vi "mmWave RX driver (FPGA).vi"() -> ()   [LabVIEW 2019]
uses:
  SubVIs/Sync/Sync Control.ctl
  SubVIs/Sync/Sync Measurements.ctl
  <instrlib>/_niInstr/DSP/v1/Shared/Public/IQ Impairments.ctl
  <instrlib>/_niInstr/DSP/v1/Shared/Public/Filter Coefficients.ctl
  Host/SubVIs/Low-level/TypeDefs/Gain Setting.ctl
  <instrlib>/niMmWave/ni3620/Config/v1/FPGA/Public/Typedefs/TX1 RX1 Port.ctl
  SubVIs/Utility/FPGA driver trigger source.ctl
  SubVIs/Utility/FPGA driver trigger destination.ctl
  <instrlib>/FlexRIO/DRAM FIFO/v2/FPGA/DRAM FIFO/DRAM FIFO Status.ctl
  <vilib>/Platform/TimedLoop/XDataNode/timing_clust.ctl
  <vilib>/Platform/TimedLoop/XDataNode/nitl_modes.ctl
  <vilib>/Platform/TimedLoop/XDataNode/wakeup.ctl
  <instrlib>/FlexRIO/DRAM FIFO/v2/FPGA/DRAM FIFO/FIFO Depth.ctl
  <instrlib>/FlexRIO/DRAM FIFO/v2/FPGA/DRAM FIFO/dynamic arbitration select.ctl
  <instrlib>/FlexRIO/DRAM FIFO/v2/FPGA/DRAM FIFO/Private/DRAM FIFO U512/Create 512x1 DRAM FIFO.vi
  <vilib>/rvi/Emulation/niFpgaSctlEmulationGetInTimedLoop.vi
  <vilib>/rvi/Emulation/niFpgaEmulationReportErrorSimple.vi
  <vilib>/rvi/Emulation/niFpgaGetClockAttributes.vi
  <vilib>/rvi/Emulation/niFpgaCriticalErrorInLSC.vi
  <vilib>/rvi/Emulation/niFpgaProcessEmulError.vi
  <vilib>/rvi/interface/RandomDataEmulation/nirviRandomDataMultiElementFPGAFIFO.vi
  <instcachedir>/0/nirviRandomDataMultiElementFPGAFIFO_1ED88BA00AC641F388A9B1FAA20E354D.lvgen/nirviRandomDataMultiElementFPGAFIFO_1ED88BA00AC641F388A9B1FAA20E354D_003.vi
  <vilib>/rvi/interface/RandomDataEmulation/niFpgaRandomDataHandleErrors.vi
  <vilib>/rvi/eio/common/nirviEmuTemplateMethod_errors.vi
  <instrlib>/_niInstr/Basic Elements/v1/FPGA/Private/Count Up U16.vi
  SubVIs/Misc/Globals.vi
  <instrlib>/_niInstr/Basic Elements/v1/FPGA/Private/Count Down U32.vi
  <instrlib>/FlexRIO/DRAM FIFO/v2/FPGA/DRAM FIFO/Pack Boolean Array.vi
  <instrlib>/_niInstr/Data Formatting/v1/FPGA/Private/Convert/FXP(+-,12,1) array to Boolean Array.vi
  <vilib>/rvi/DataTransferAndStorage/Container/Common/niFpgaContainerGetUniqueNameForEmu.vi
  <vilib>/rvi/DataTransferAndStorage/Container/Common/niFpgaContainerSetEmuInfo.vi
  <vilib>/rvi/eio/common/nirviEmuReportErrorAndStop.vi
  <vilib>/rvi/Emulation/niFpgaEmulationIsFPGAContextNoSignature.vi
  <vilib>/rvi/errors/niFpgaSetErrorForExecOnDevCompSimple.vi
  <vilib>/rvi/FIFO/Fifo_Resource/nirvififoEmulationSetSize.vi
  <vilib>/rvi/FIFO/Fifo_Resource/nirviFifoEmulationQueueMgr.vi
  <instcachedir>/0/nirviFifoEmulationQueueMgr_E5CAEC123FF24DC58D834DCA3CDAA9B5.lvgen/nirviFifoEmulationQueueMgr_E5CAEC123FF24DC58D834DCA3CDAA9B5_008.vi
  <vilib>/Utility/error.llb/Clear Errors.vi
  <vilib>/rvi/FIFO/Fifo_Resource/nirvififoEmulationCreateLock.vi
  <vilib>/rvi/FIFO/Fifo_Resource/nirvififoEmulationObtainLock.vi
  <vilib>/rvi/FIFO/Fifo_Resource/nirvififoEmulationReleaseLock.vi
  <vilib>/rvi/occurrence/nirviWaitOnOccurrenceBase.vi
  <vilib>/rvi/errors/nirviReportUnexpectedCaseInternalError.vi
  <vilib>/rvi/errors/nirviReportUnexpectedCaseInternalError (U32).vi
  <vilib>/rvi/FIFO/Fifo_Resource/nirvififoEmulationDetermineInputValidOut.vi
  <vilib>/Platform/TimedLoop/XDataNode/XDataNode.xnode
  <vilib>/rvi/DataTransferAndStorage/Container/XNode/niFpgaContainer.xnode
  <vilib>/rvi/interface/RandomDataEmulation/nirviRandomDataFpgaMultiElementTemplate.vi
  <vilib>/eio/EIONode/EIONode.xnode
  <vilib>/eio/EIOMethodNode/EIOMethodNode.xnode
  <vilib>/rvi/LocalResourceManager/LocalResourceManager.xnode
  <vilib>/rvi/FIFO/Fifo_Resource/nirvififoEmulationRead.vi
  <vilib>/rvi/FIFO/Fifo_Resource/nirvififoEmulationWrite.vi
  <vilib>/Platform/TimedLoop/XDataNode/XDNodeRunTimeDep.lvlib
  <instrlib>/_niInstr/Basic Elements/v1/FPGA/niInstr Basic Elements v1 FPGA.lvlib
  <instrlib>/niMmWave/ni3620/Config/v1/FPGA/niMmWave Config v1 FPGA.lvlib
  SubVIs/Utility/FPGA Utility.lvlib
  <instrlib>/FlexRIO/DRAM FIFO/v2/FPGA/DRAM FIFO/DRAM FIFO v2 FPGA.lvclass
  <instrlib>/_niInstr/Data Formatting/v1/FPGA/niInstr Data Formatting v1 FPGA.lvlib
  <instrlib>/FlexRIO/DRAM FIFO/v2/FPGA/DRAM FIFO/Private/DRAM FIFO U512/DRAM FIFO U512 v2 FPGA.lvclass
  <instrlib>/_niInstr/DSP/v1/Shared/niInstr DSP v1 Shared.lvlib
panel:
  out "dram.in fifo max":u32
  out "dram.highwater":u32
  out "dram.reset in progress?":bool
  in  "dram.reset":bool
  out "dram.status":T1
  out "dram.overflow":bool
  in  "dram.flush":bool
  out "acquisition active":bool
  out "aurora.data":u16
  out "aurora.trig count":u16
  out "pxi.trig count":u16
  out "aurora.tx val":u16
  in  "trig.pxi dst":i32
  in  "trig.export":T2
  in  "trig.export dur":u32
  in  "trig.source":T3
  out "debug.trig.count":u16
  in  "trig.delay":u16
  in  "trig.pxi src":i32
  in  "sync.master reset listen":bool
  in  "sync.counter reset enable":bool
  in  "20 kHz tclk parameters":T4
  out "tclk value":u16
  in  "gain ranging.enable port config":bool
  out "port 5.debug info":T5
  out "port 5.rx fifo overflow":bool
  in  "port 5.rx fifo overflow clear":bool
  in  "aurora.read port 5":bool
  out "port 4.rx fifo overflow":bool
  in  "port 4.rx fifo overflow clear":bool
  out "port 4.debug info":T5
  in  "aurora.read port 4":bool
  in  "gain ranging.enable coarse gain ranging":bool
  in  "gain ranging.enable fine gain ranging":bool
  in  "gain ranging.coarse gain values":fxp<+/-,16,12>[](array[numeric])=[0.0, 0.0, 0.0, 0.0]
  in  "table info":T6
  in  "gain ranging.manual setting":T9
  in  "gain ranging.setting list step":T10
  in  "gain ranging.enable":bool
  in  "gain ranging.dwell time (cycles)":u32=4800
  in  "rxjesd.control":T11
  out "rxjesd.status":T12
  in  "filter.enable":bool
  in  "filter.coefficients":T13
  in  "cal.correction":T15={"sample delay"={"I delay"=0.0, "Q delay"=0.0}, "fractional delay"={"enable"=FALSE, "coef write"=FALSE, "coef data"=0.0}, "impairments"={"inline gain I"=0.9999923706054688, "inline gain Q"=0.9999923706054688, "cross gain I"=0.0, "cross gain Q"=0.0, "pre-gain offset I"=0.0, "pre-gain offset Q"=0.0, "post-gain offset I"=0.0, "post-gain offset Q"=0.0}, "iq inversion"={"invert I"=FALSE, "invert Q"=FALSE}}
  out "sync.measurements":T16
  in  "sync.parameters":T18
  in  "acq.length":u32=1024
  out "aurora.fifo 1 overflow":bool
  in  "aurora.reset trigger":bool=TRUE
  out "aurora.fifo 0 overflow":bool
  in  "aurora.write":bool
  in  "aurora.fifo overflow clear":bool
  out "clocks valid":bool[](array[boolean])
  in  "cal.acquisition":T19={"acq length"=1024, "trigger type"=enum."software", "software trigger"=FALSE, "reset trigger detect"=FALSE}
  in  "sync.use synced trigger":bool
  in  "sync.trigger":bool
  # "DRAM and ACQUISITION"
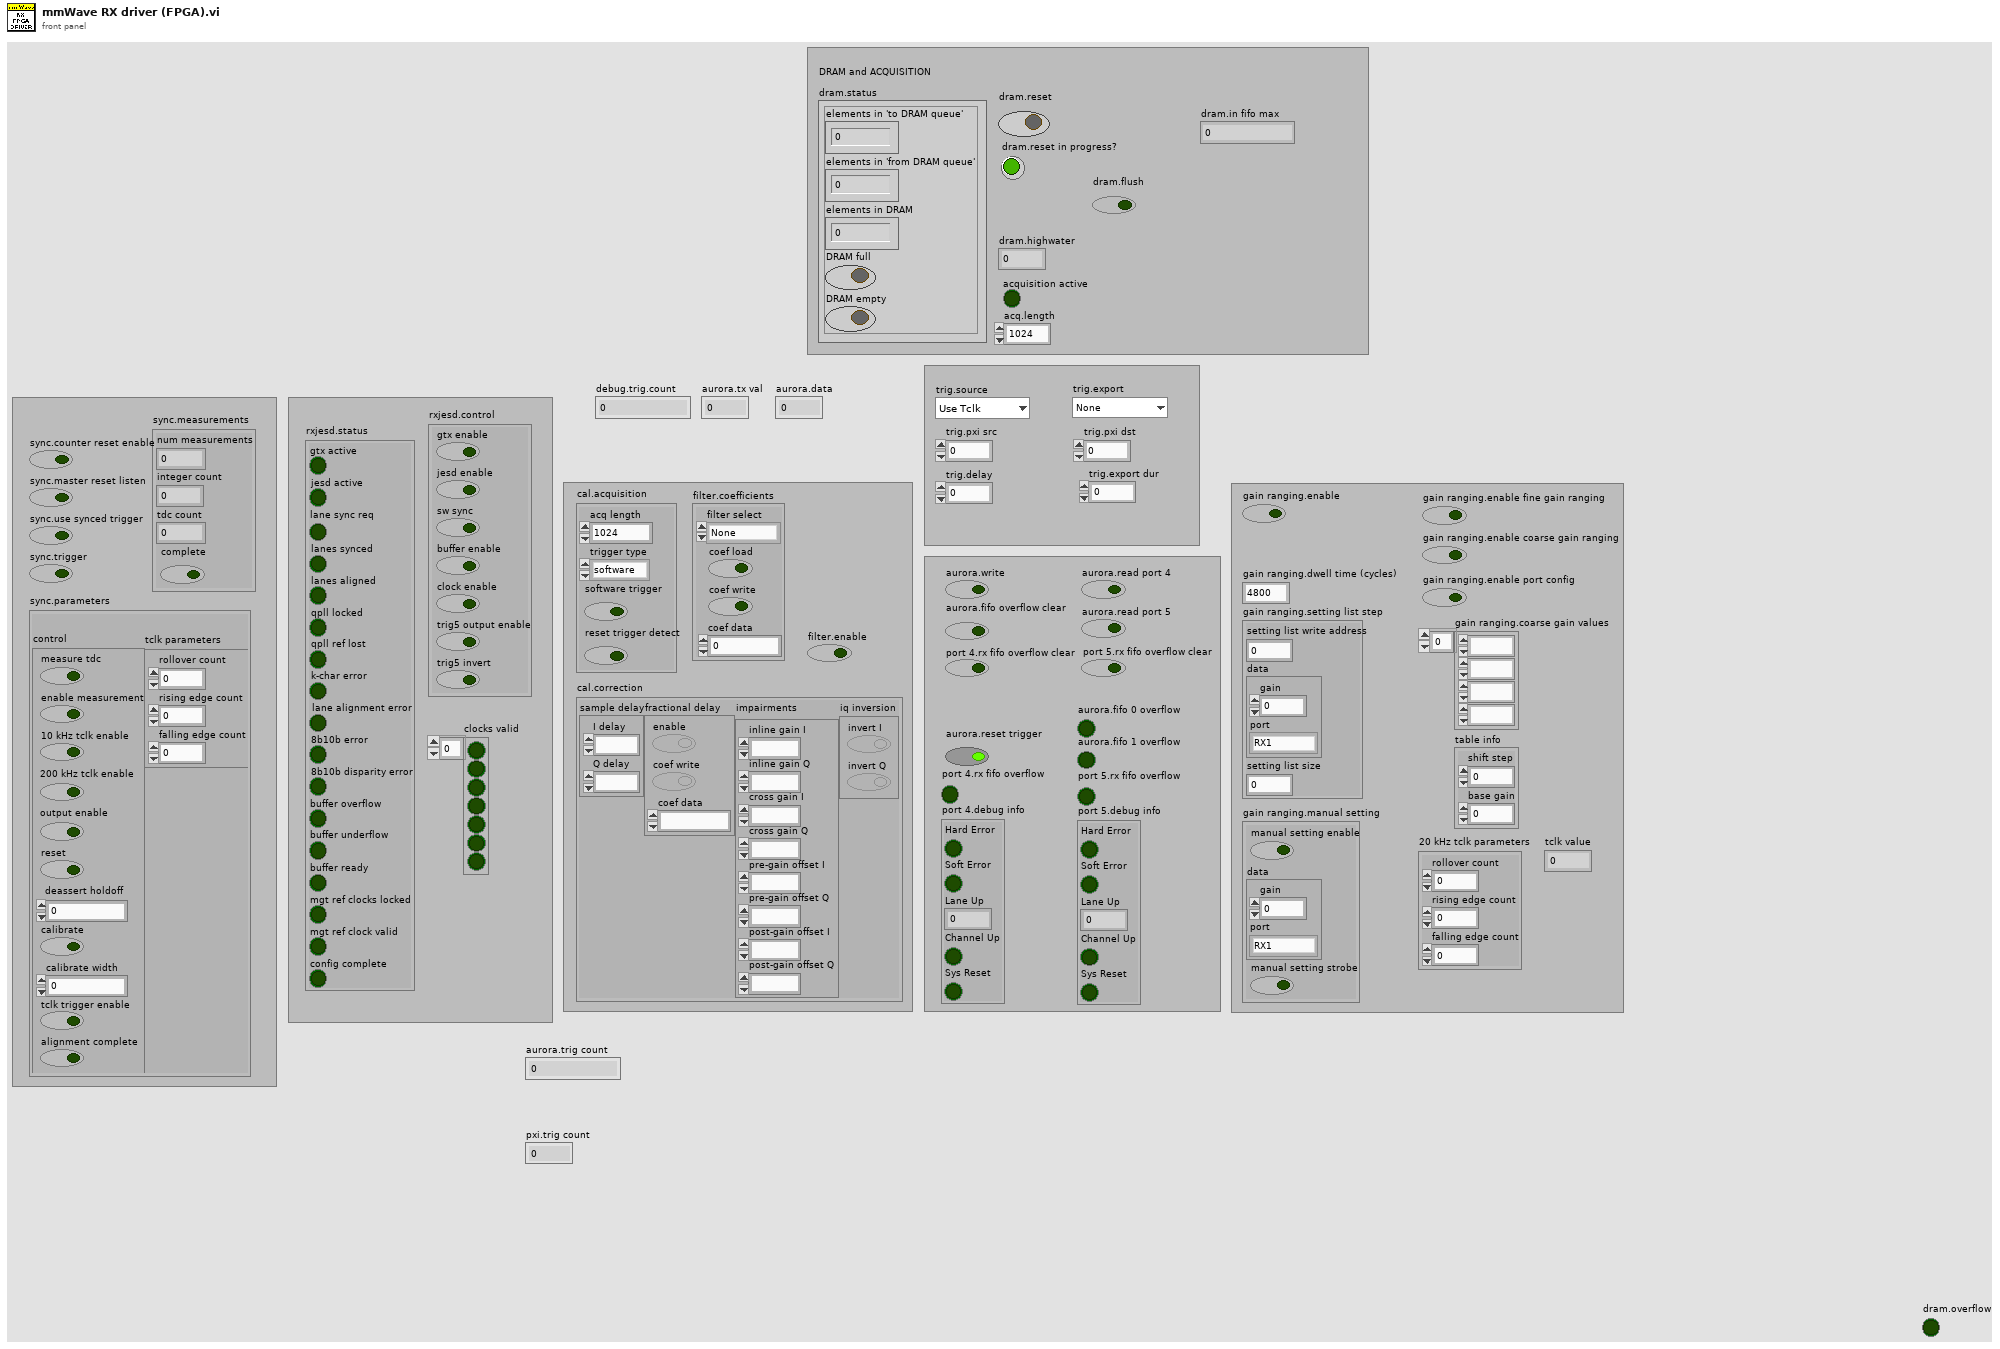
[diagram p1: front panel]
types:
  T1 = typedef "DRAM FIFO v2 FPGA.lvclass/DRAM FIFO Status.ctl" = cluster{"elements in 'to DRAM queue'":u32, "elements in 'from DRAM queue'":u32, "elements in DRAM":u32, "DRAM full":bool, "DRAM empty":bool}
  T2 = typedef "FPGA Utility.lvlib/FPGA driver trigger destination.ctl" = enum16{"None", "Source trig", "Synced trig", "Delayed sync"}
  T3 = typedef "FPGA Utility.lvlib/FPGA driver trigger source.ctl" = enum16{"Use Tclk", "PXI_Trig", "Aurora RX trig"}
  T4 = cluster{"rollover count":u16, "rising edge count":u16, "falling edge count":u16}
  T5 = cluster{"Hard Error":bool, "Soft Error":bool, "Lane Up":fxp<+,4,4>, "Channel Up":bool, "Sys Reset":bool}
  T6 = cluster{"shift step":i16, "base gain":fxp<+/-,16,12>}
  T7 = typedef "gain setting.ctl" = cluster{"gain":fxp<+/-,16,12>, "port":T8}
  T8 = typedef "TX1 RX1 Port.ctl" = enum8{"RX1", "TX1/RX2"}
  T9 = cluster{"manual setting enable":bool, "data":T7, "manual setting strobe":bool}
  T10 = cluster{"setting list write address":u32, "data":T7, "setting list size":u16}
  T11 = cluster{"gtx enable":bool, "jesd enable":bool, "sw sync":bool, "buffer enable":bool, "clock enable":bool, "trig5 output enable":bool, "trig5 invert":bool}
  T12 = cluster{"gtx active":bool, "jesd active":bool, "lane sync req":bool, "lanes synced":bool, "lanes aligned":bool, "qpll locked":bool, "qpll ref lost":bool, "k-char error":bool, "lane alignment error":bool, "8b10b error":bool, "8b10b disparity error":bool, "buffer overflow":bool, "buffer underflow":bool, "buffer ready":bool, "mgt ref clocks locked":bool, "mgt ref clock valid":bool, "config complete":bool}
  T13 = typedef "niInstr DSP v1 Shared.lvlib/Filter Coefficients.ctl" = cluster{"filter select":enum8{"None", "I Inline", "I Cross", "Q Cross", "Q Inline"}, "coef load":bool, "coef write":bool, "coef data":fxp<+/-,18,1>}
  T14 = typedef "niInstr DSP v1 Shared.lvlib/IQ Impairments.ctl" = cluster{"inline gain I":fxp<+/-,18,1>, "inline gain Q":fxp<+/-,18,1>, "cross gain I":fxp<+/-,18,1>, "cross gain Q":fxp<+/-,18,1>, "pre-gain offset I":fxp<+/-,18,1>, "pre-gain offset Q":fxp<+/-,18,1>, "post-gain offset I":fxp<+/-,18,1>, "post-gain offset Q":fxp<+/-,18,1>}
  T15 = cluster{"sample delay":cluster{"I delay":fxp<+,13,13>, "Q delay":fxp<+,13,13>}, "fractional delay":cluster{"enable":bool, "coef write":bool, "coef data":fxp<+/-,18,1>}, "impairments":T14, "iq inversion":cluster{"invert I":bool, "invert Q":bool}}
  T16 = typedef "Sync Measurements.ctl" = cluster{"num measurements":u16, "integer count":u16, "tdc count":u16, "complete":bool}
  T17 = typedef "Sync Control.ctl" = cluster{"measure tdc":bool, "enable measurement":bool, "10 kHz tclk enable":bool, "200 kHz tclk enable":bool, "output enable":bool, "reset":bool, "deassert holdoff":u8, "calibrate":bool, "calibrate width":u8, "tclk trigger enable":bool, "alignment complete":bool}
  T18 = cluster{"control":T17, "tclk parameters":cluster{"rollover count":u16, "rising edge count":u16, "falling edge count":u16}}
  T19 = cluster{"acq length":u16, "trigger type":enum16{"software", "external", "rising zero", "falling zero"}, "software trigger":bool, "reset trigger detect":bool}
  T20 = typedef "DRAM FIFO v2 FPGA.lvclass/FIFO Depth.ctl" = u8
  T21 = cluster{"m_axis_tvalid":refnum<k21>, "m_axis_tdata_0":refnum<k21>, "m_axis_tdata_1":refnum<k21>, "m_axis_tdata_2":refnum<k21>, "m_axis_tdata_3":refnum<k21>}
  T22 = cluster{"s_axis_tvalid":refnum<k21>, "s_axis_tdata_0":refnum<k21>, "s_axis_tdata_1":refnum<k21>, "s_axis_tdata_2":refnum<k21>, "s_axis_tdata_3":refnum<k21>, "s_axis_tready":refnum<k21>}
  T23 = typedef "XDNodeRunTimeDep.lvlib/timing_clust.ctl" = cluster{"Expected End [f-1]":u64, "Actual End [f-1]":u64, "Finished Late? [f-1]":bool, "Expected End [i-1]":u64, "Actual End [i-1]":u64, "Finished Late? [i-1]":bool, "Expected Start [i]":u64, "Actual Start [i]":u64, "Expected Start [f]":u64, "Actual Start [f]":u64, "Source Name":string, "Structure Name":string, "Period":i64, "Deadline":i64, "Offset":i64, "Start":i64, "Priority":i32, "Timeout":i32, "Mode":T24, "Wakeup Reason":T25, "Error":errorcluster, "Source Type":string, "Secondary Source Type":string, "Global End Time":u64, "Global Start Time":u64, "Frame Duration":u64, "Iteration Duration":u64, "Assigned CPU":i32, "I/O Scan Engine Mode":u32}
  T24 = typedef "XDNodeRunTimeDep.lvlib/nitl_modes.ctl" = enum32{"No Change", "Process missed periods, maintain original phase", "Discard missed periods, maintain original phase", "Process missed periods, ignore original phase", "Discard missed periods, ignore original phase"}
  T25 = typedef "XDNodeRunTimeDep.lvlib/wakeup.ctl" = enum32{"Normal", "Aborted", "Asynchronous wakeup", "Timing source error", "Timed loop error", "Timeout"}
  T26 = typedef "Sync Resources.ctl" = cluster{"tdc assert":refnum<k21>, "tdc deassert":refnum<k21>, "tdc count":refnum<k21>, "control":refnum<k21>, "integer count":refnum<k21>}
  T27 = typedef "DRAM FIFO v2 FPGA.lvclass/dynamic arbitration select.ctl" = enum16{"none", "dynamic (priority writes)", "dynamic (priority reads)"}
  T28 = cluster{"disable TClk measure":bool, "output enable":bool, "output value":bool}
  T29 = typedef "niInstr DSP v1 Shared.lvlib/IQ Data.ctl" = cluster{"I":fxp<+/-,18,1>, "Q":fxp<+/-,18,1>, "overflow":bool}
  T30 = typedef "AXI4-Stream Reader FXP64x4 Resources.ctl" = cluster{"AXI4-Stream Reader Resources":cluster{"Use TREADY":bool, "Use TLAST":bool, "TLAST":refnum<k21>, "TREADY":refnum<k21>, "TVALID":refnum<k21>, "Use TKEEP":bool, "Use TSTRB":bool, "Use TUSER":bool}, "TDATA Resources":cluster{"TDATA_0":refnum<k21>, "TDATA_1":refnum<k21>, "TDATA_2":refnum<k21>, "TDATA_3":refnum<k21>}, "TKEEP":refnum<k21>, "TSTRB":refnum<k21>}
  T31 = typedef "AXI4-Stream Writer FXP64x4 Resources.ctl" = cluster{"Writer Resources":cluster{"Use TREADY":bool, "Use TLAST":bool, "TLAST":refnum<k21>, "TREADY":refnum<k21>, "TVALID":refnum<k21>, "Use TSTRB":bool, "Use TKEEP":bool, "Use TUSER":bool}, "TDATA Resources":cluster{"TDATA_0":refnum<k21>, "TDATA_1":refnum<k21>, "TDATA_2":refnum<k21>, "TDATA_3":refnum<k21>}, "TKEEP":refnum<k21>, "TSTRB":refnum<k21>}
  T32 = cluster{"Hard Error":refnum<k21>, "Soft Error":refnum<k21>, "Lane Up":refnum<k21>, "Channel Up":refnum<k21>, "Sys Reset":refnum<k21>}
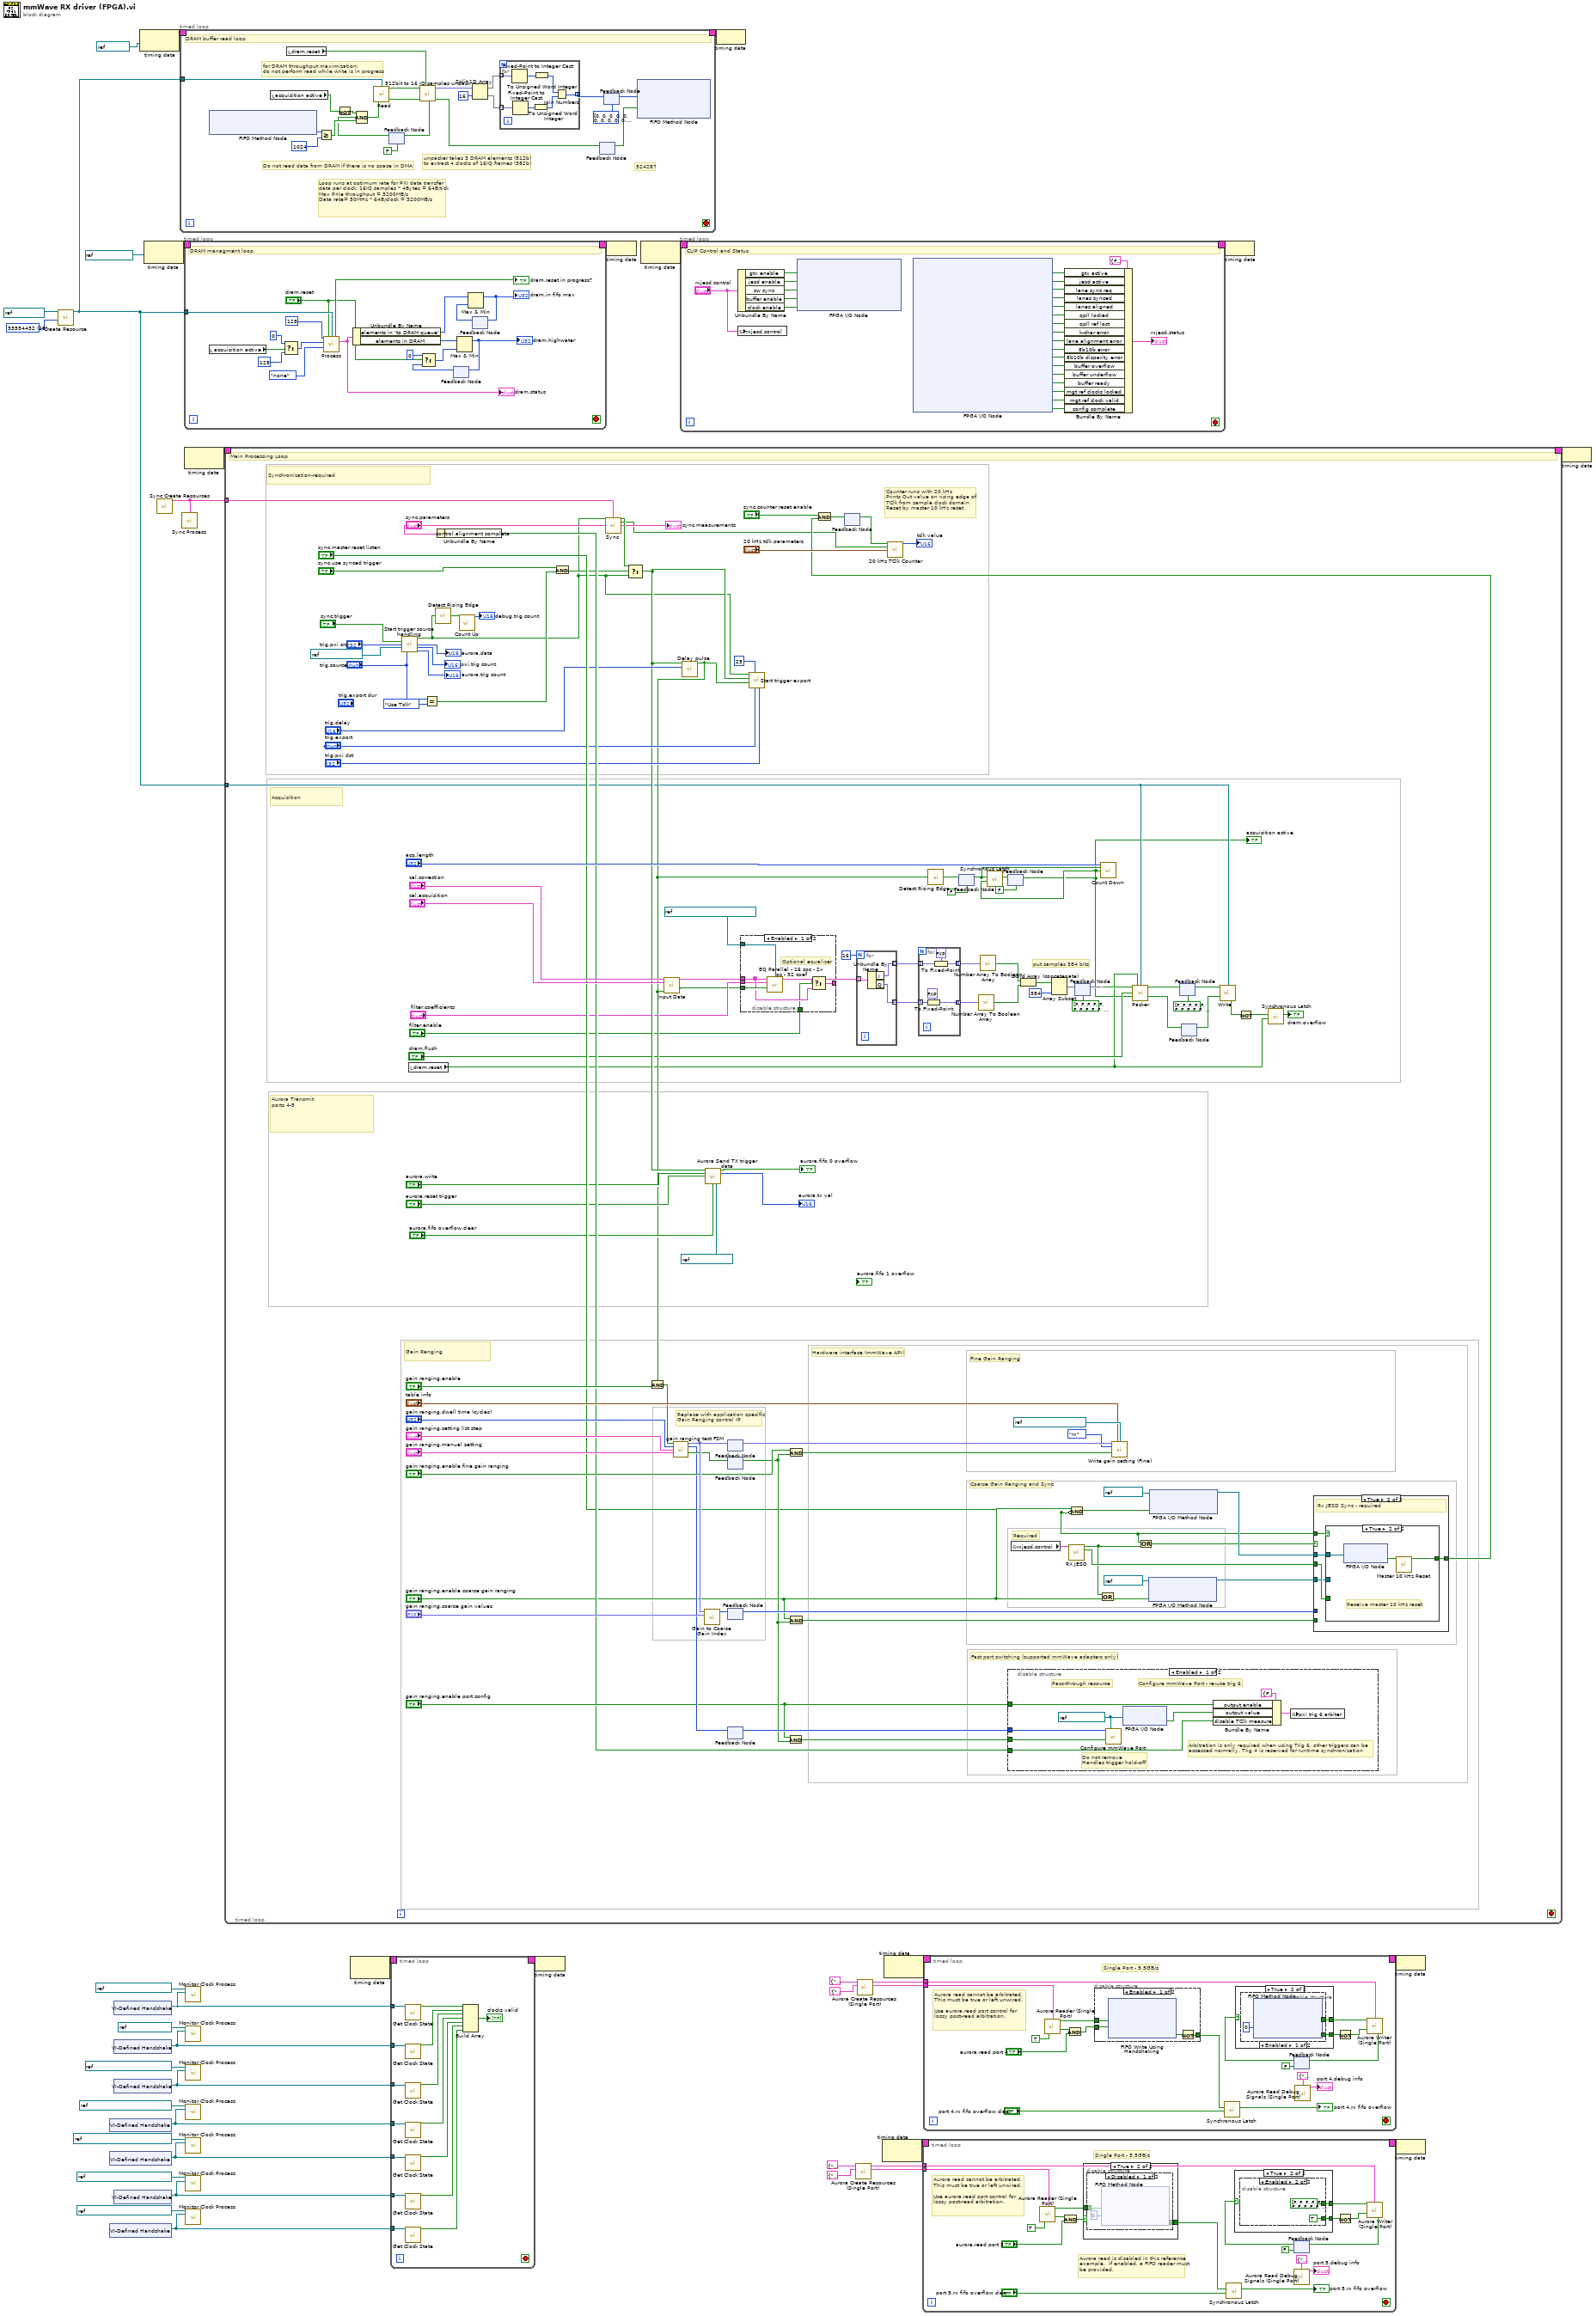
[diagram p0: block diagram]
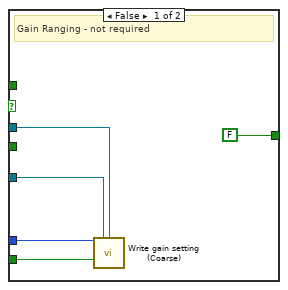
[diagram p3: hidden frame]
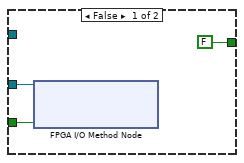
[diagram p4: hidden frame]
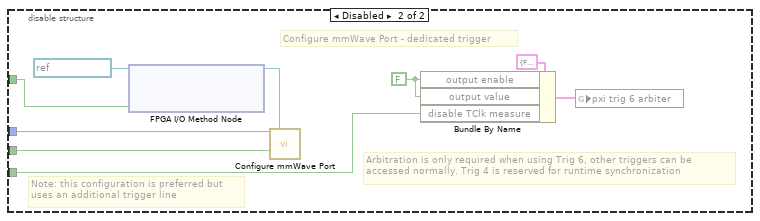
[diagram p5: hidden frame]
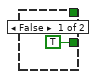
[diagram p6: hidden frame]
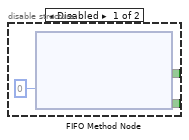
[diagram p7: hidden frame]
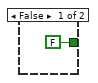
[diagram p8: hidden frame]
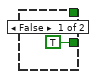
[diagram p11: hidden frame]
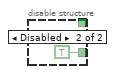
[diagram p12: hidden frame]
diagram:
  w1 = T20 25 items=["4"=2, "8"=3, "16"=4, "32"=5, "64"=6, "128"=7, "256"=8, "512"=9, "1024"=10, "2048"=11, "4096"=12, "8192"=13, "16384"=14, "32768"=15, "65536"=16, "131072"=17, "262144"=18, "524288"=19, "1048576"=20, "2097152"=21, "4194304"=22, "8388608"=23, "16777216"=24, "33554432"=25, "67108864"=26, "134217728"=27, "268435456"=28, "536870912"=29, "1073741824"=30, "2147483648"=31, "4294967296"=32] ("actual # of DRAM elements")
  n1 = call-poly <instrlib>:"Create Resource.vi"("actual # of DRAM elements"=w1, "memory refnum"=refnum<k21> "RX memo") -> ("DRAM FIFO ref out"=w2:refnum<class "DRAM FIFO v2 FPGA.lvclass">)  [unwired: 9 in]
  n2 = xnode "VI-Defined Handshake"() -> ("Handshake Out"=w19:refnum<k21>)
  n3 = xnode "VI-Defined Handshake"() -> ("Handshake Out"=w20:refnum<k21>)
  n4 = xnode "VI-Defined Handshake"() -> ("Handshake Out"=w27:refnum<k21>)
  n5 = xnode "VI-Defined Handshake"() -> ("Handshake Out"=w34:refnum<k21>)
  n6 = xnode "VI-Defined Handshake"() -> ("Handshake Out"=w33:refnum<k21>)
  n7 = xnode "VI-Defined Handshake"() -> ("Handshake Out"=w29:refnum<k21>)
  n8 = xnode "VI-Defined Handshake"() -> ("Handshake Out"=w30:refnum<k21>)
  n9 = node-c288(refnum<k21> "50MHz" ("Source Name")) -> (w5:T23)
  n10 = node-c288(refnum<k21> "DRAM Clock" ("Source Name")) -> (w8:T23)
  n11 = call "Sync Create Resources.vi"() -> ("sync.resources"=w38:T26)  [unwired: 15 in]
  n12 = timed-loop {
    timing: w5 -> [_]
    timing-out: [_] -> w4
    tunnel: w2 -> [w46]
    stop <- _ stop-if-true
    # "524287"
    # "unpacker takes 3 DRAM elements (512b)\nto extract 4 clocks of 16IQ frames (382b)"
    # "Do not read data from DRAM if there is no space in DMA"
    # "for DRAM throughput maximization:\ndo not perform read while write is in progress"
    # "Loop runs at optimum rate for PXI data transfer\ndata per clock: 16IQ samples * 4Bytes = 64B/tick\nMax PXIe throughput = 3200MB/s\nData rate= 50MHz * 64B/clock = 3200MB/s"
    # "DRAM buffer read loop"
    n13 = xnode ("FIFO Method Node")() -> ("Number of Elements to Write"=w57:u32)  [unwired: 1 in, 1 out]
    n14 = local read "acquisition active"() -> (w45:bool)
    n15 = local read "dram.reset"() -> (w43:bool)
    n16 = Greater Or Equal?(x=w57, y=u32 1024) -> (x >= y?=w59:bool)
    n17 = Not(x=w45) -> (.not. x?=w48:bool)
    n18 = feedback #1(FALSE ("ready for input")) -> (w49:bool)
    n19 = Compound Arithmetic op=AND(w48, w49, w59) -> (w50:bool)
    n20 = call <instrlib>:"Read.vi"("DRAM FIFO ref in"=w46, "ready for output"=w50) -> ("element"=w51:bool[], "output valid"=w52:bool)  [unwired: 12 in]
    n21 = call "512bit to 16 IQ samples unpack.vi"("reset"=w43, "input valid"=w52, "data in"=w51) -> ("output valid"=w63:bool, "data out"=w54:fxp<+/-,12,1>[], "ready for input"=w53:bool)  [unwired: 6 in]
    n22 = feedback-in #1(w53) -> ()
    n23 = Split 1D Array(array=w54, index=16) -> (first subarray=w55:fxp<+/-,12,1>[], second subarray=w56:fxp<+/-,12,1>[])
    n24 = for {
      tunnel: w55 -> [w71] mode=indexing
      tunnel: w56 -> [w70] mode=indexing
      tunnel: [w67] -> w60 mode=indexing
      n25 = Fixed-Point to Integer Cast(1:w71) -> (0:w66:i16)
      n26 = Fixed-Point to Integer Cast(1:w70) -> (0:w65:i16)
      n27 = To Unsigned Word Integer(number=w65) -> (unsigned 16bit integer=w68:u16)
      n28 = To Unsigned Word Integer(number=w66) -> (unsigned 16bit integer=w69:u16)
      n29 = Join Numbers(hi=w69, lo=w68) -> ((hi.lo)=w67:u32)
    }
    n30 = feedback #2() -> (w64:bool)  [unwired: 1 in]
    n31 = feedback-in #2(w63) -> ()
    n32 = feedback #3(u32[] [0, 0, 0, 0, 0, 0, 0, 0, 0, 0, 0, 0, 0, 0, 0, 0]) -> (w61:u32[])
    n33 = feedback-in #3(w60) -> ()
    n34 = xnode ("FIFO Method Node")("Element"=w61, "Input Valid"=w64) -> ()  [unwired: 1 in, 2 out]
  }
  n35 = call "Sync Process.vi"("sync.resources"=w38) -> ()  [unwired: 15 in]
  n36 = timed-loop {
    timing: w8 -> [_]
    timing-out: [_] -> w7
    tunnel: w2 -> [w85]
    stop <- _ stop-if-true
    # "DRAM managment loop"
    n37 = local read "acquisition active"() -> (w78:bool)
    n38 = Select(t=u16 0, s=w78, f=u16 128 ("read grant time (clock ticks)")) -> (s? t:f=w76:u16)
    n39 = call <instrlib>:"Process.vi"("write grant time (clock ticks)"=u16 128, "reset DRAM"="dram.reset", "DRAM FIFO ref in"=w85, "read grant time (clock ticks)"=w76, "dynamic arbitration"=dynamic_arbitration_select."none") -> ("reset in progress?"=→"dram.reset in progress?":bool, "status"=w88:T1)  [unwired: 9 in]
    "dram.status" <- w88
    n40 = Unbundle By Name(w88) -> ("elements in 'to DRAM queue'"=w80:u32, "elements in DRAM"=w87:u32)
    n41 = feedback #4() -> (w83:u32)  [unwired: 1 in]
    n42 = Select(t=u32 0, s="dram.reset", f=w83) -> (s? t:f=w81:u32)
    n43 = Max & Min(x=w87, y=w81) -> (max(x,y)=w86:u32)  [unwired: 1 out]
    "dram.highwater" <- w86
    n44 = feedback-in #4(w86) -> ()
    n45 = feedback #5() -> (w79:u32)  [unwired: 1 in]
    n46 = Max & Min(x=w80, y=w79) -> (max(x,y)=w74:u32)  [unwired: 1 out]
    "dram.in fifo max" <- w74
    n47 = feedback-in #5(w74) -> ()
  }
  n48 = node-c288() -> (w40:T23)  [unwired: 1 in]
  n49 = call "Monitor Clock Process.vi"("clock name"=refnum<k21> "40 MHz Onboard Clock", "handshake"=w34) -> ()  [unwired: 14 in]
  n50 = call "Monitor Clock Process.vi"("clock name"=refnum<k21> "100 MHz Clock", "handshake"=w33) -> ()  [unwired: 14 in]
  n51 = call "Monitor Clock Process.vi"("clock name"=refnum<k21> "7902R IO Socket\\SampleClk", "handshake"=w29) -> ()  [unwired: 14 in]
  n52 = call "Monitor Clock Process.vi"("clock name"=refnum<k21> "7902R IO Socket\\SampleClkx2", "handshake"=w19) -> ()  [unwired: 14 in]
  n53 = call "Monitor Clock Process.vi"("clock name"=refnum<k21> "7902R IO Socket\\SampleClkDiv2", "handshake"=w20) -> ()  [unwired: 14 in]
  n54 = call "Monitor Clock Process.vi"("clock name"=refnum<k21> "7902R IO Socket\\Port4_UserClk", "handshake"=w30) -> ()  [unwired: 14 in]
  n55 = call "Monitor Clock Process.vi"("clock name"=refnum<k21> "7902R IO Socket\\Port5_UserClk", "handshake"=w27) -> ()  [unwired: 14 in]
  n56 = timed-loop {
    timing: w40 -> [_]
    timing-out: [_] -> w39
    tunnel: w38 -> [w196]
    tunnel: w2 -> [w110]
    stop <- _ stop-if-true
    # "put samples 384 bits"
    # "Counter runs with 20 kHz\nPrints Out value on rising edge of \nTClk from sample clock domain\nReset by master 10 kHz reset"
    # "Replace with application specific Gain Ranging control IP"
    # "Fast port switching (supported mmWave adapters only)"
    # "Coarse Gain Ranging and Sync"
    # "Fine Gain Ranging"
    # "Hardware interface (mmWave API)"
    # "Gain Ranging"
    # "Aurora Transmit\nports 4-5"
    # "Acquisition"
    # "Synchronization-required"
    # "Required"
    # "Main Processing Loop"
    n57 = call "Start trigger source handling.vi"("sync.trigger"="sync.trigger", "trig.pxi trig src"="trig.pxi src", "Refnum in"=refnum<k21> "aurora rx fifo 0" ("FIFO In"), "trig.source"="trig.source") -> ("trigger"=w126:bool, "aurora.data"=→"aurora.data":u16, "pxi.trig count"=→"pxi.trig count":u16, "aurora.trig count"=→"aurora.trig count":u16)  [unwired: 8 in]
    n58 = local read "dram.reset"() -> (w100:bool)
    n59 = Equal?(x="trig.source", y=FPGA_driver_trigger_source."Use Tclk") -> (x = y?=w128:bool)
    n60 = call <instrlib>:"Detect Rising Edge.vi"("signal"=w126) -> ("edge detected"=w148:bool)  [unwired: 14 in]
    n61 = Unbundle By Name("sync.parameters") -> ("control.alignment complete"=w162:bool)
    n62 = call-poly <instrlib>:"Count Up.vi"("increment"=w148) -> ("count out"=→"debug.trig.count":u16)  [unwired: 14 in]
    n63 = And(x="sync.use synced trigger", y=w128) -> (x .and. y?=w129:bool)
    n64 = call "Sync.vi"("trigger"=w126, "sync.resources"=w196, "sync.parameters"="sync.parameters") -> ("synced trigger"=w197:bool, "tclk"=w153:bool, "sync measurements"=→"sync.measurements":T16)  [unwired: 10 in]
    n65 = Select(t=w197, s=w129, f=w126) -> (s? t:f=w140:bool)
    n66 = call "Delay pulse.vi"("delay"="trig.delay", "signal in"=w140) -> ("delayed rising edge"=w125:bool)  [unwired: 9 in]
    n67 = And(x=w125, y="gain ranging.enable") -> (x .and. y?=w177:bool)
    n68 = call "Input Data.vi"("cal parameters"="cal.correction", "acq parameters"="cal.acquisition", "external trigger"=w125) -> ("adc data"=w98:T29[], "output valid"=w94:bool)  [unwired: 11 in]
    n69 = call "gain ranging test FSM.vi"("gain ranging.start sequence"=w177, "gain ranging.dwell time (cycles)"="gain ranging.dwell time (cycles)", "gain ranging.gain setting list"="gain ranging.setting list step", "gain ranging.manual request"="gain ranging.manual setting") -> ("gain ranging.gain setting"=w186:fxp<+/-,16,12>, "gain ranging.TX1/RX1 Port Value"=w179:T8, "gain ranging.gain setting valid"=w181:bool)  [unwired: 8 in, 1 out]
    n70 = call "Gain to Coarse Gain Index.vi"("gain setting"=w186, "coarse gain values"="gain ranging.coarse gain values") -> ("coarse gain index"=w184:u32)  [unwired: 13 in]
    n71 = call "Aurora Send TX trigger data.vi"("start trigger"=w140, "aurora.write"="aurora.write", "aurora.reset trigger"="aurora.reset trigger", "clear overflow"="aurora.fifo overflow clear", "aurora tx fifo"=refnum<k21> "aurora tx fifo 0" ("FIFO In")) -> ("tx overflow latch"=→"aurora.fifo 0 overflow":bool, "trig count"=→"aurora.tx val":u16)  [unwired: 9 in]
    n72 = feedback #6() -> (w185:fxp<+/-,16,12>)  [unwired: 1 in]
    n73 = feedback-in #6(w186) -> ()
    n74 = feedback #7() -> (w167:bool)  [unwired: 1 in]
    n75 = feedback-in #7(w181) -> ()
    n76 = feedback #8() -> (w170:u32)  [unwired: 1 in]
    n77 = feedback-in #8(w184) -> ()
    n78 = feedback #9() -> (w175:T8)  [unwired: 1 in]
    n79 = feedback-in #9(w179) -> ()
    n80 = disable-structure shown="Enabled" {
      disable-tunnel: w94 -> [w211 _]
      disable-tunnel: [w209 w212] -> w97
      disable-tunnel: w98 -> [w208 w212]
      disable-tunnel: "filter.coefficients" -> [w207 _]
      disable-tunnel: "filter.enable" -> [w206 _]
      disable-tunnel: refnum<k21> "7902R IO Socket\\SampleClkx2" ("clock x2") -> [w205 _]
      frame Enabled {
        # "Optional equalizer"
        n81 = call "EQ Parallel - 16 spc - 2x oc - 32 coef.vi"("data in"=w208, "clock x2"=w205, "filter coefficients"=w207, "input valid"=w211) -> ("data out"=w210:T29[])  [unwired: 9 in, 2 out]
        n82 = Select(t=w210, s=w206, f=w208) -> (s? t:f=w209:T29[])
      }
      frame Disabled {
      }
    }
    n83 = call "Start trigger export.vi"("trig.pxi trig dst"="trig.pxi dst", "trig.export"="trig.export", "trig.dur"=u32 25, "delayed trigger"=w125, "synced trigger"=w140, "source trigger"=w126) -> ()  [unwired: 2 in, 4 out]
    n84 = And(x="gain ranging.enable port config", y=w167) -> (x .and. y?=w166:bool)
    n85 = And(x="gain ranging.enable fine gain ranging", y=w167) -> (x .and. y?=w180:bool)
    n86 = And(x="gain ranging.enable coarse gain ranging", y=w167) -> (x .and. y?=w169:bool)
    n87 = feedback #10() -> (w154:bool)  [unwired: 1 in]
    n88 = for {
      N: 16 -> [_]
      tunnel: w97 -> [w221] mode=indexing
      tunnel: [w220] -> w103 mode=indexing
      tunnel: [w219] -> w106 mode=indexing
      n89 = Unbundle By Name(w221) -> ("I"=w220:fxp<+/-,18,1>, "Q"=w219:fxp<+/-,18,1>)
    }
    n90 = call "20 kHz TClk Counter.vi"("master 10 kHz reset"=w154, "tclk"=w153, "20 kHz tclk parameters"="20 kHz tclk parameters") -> ("tclk offset value"=→"tclk value":u16)  [unwired: 12 in]
    n91 = for {
      tunnel: w103 -> [w215] mode=indexing
      tunnel: w106 -> [w217] mode=indexing
      tunnel: [w214] -> w105 mode=indexing
      tunnel: [w213] -> w104 mode=indexing
      n92 = To Fixed-Point(fixed-point type=fxp<+/-,12,1> 0.0, number=w217) -> (fixed-point=w213:fxp<+/-,12,1>)
      n93 = To Fixed-Point(fixed-point type=fxp<+/-,12,1> 0.0, number=w215) -> (fixed-point=w214:fxp<+/-,12,1>)
    }
    n94 = call <instrlib>:"Detect Rising Edge.vi"("signal"=w125) -> ("edge detected"=w108:bool)  [unwired: 14 in]
    n95 = feedback #11(FALSE ("edge detected")) -> (w200:bool)
    n96 = feedback-in #11(w108) -> ()
    n97 = call-poly <instrlib>:"Number Array To Boolean Array.vi"("data in"=w104) -> ("data out"=w121:bool[])  [unwired: 14 in]
    n98 = call-poly <instrlib>:"Number Array To Boolean Array.vi"("data in"=w105) -> ("data out"=w124:bool[])  [unwired: 14 in]
    n99 = feedback #12(FALSE ("out")) -> (w109:bool)
    "acquisition active" <- w109
    n100 = disable-structure shown="Enabled" {
      disable-tunnel: w166 -> [w243 w252]
      disable-tunnel: w175 -> [w242 w251]
      disable-tunnel: "gain ranging.enable port config" -> [w240 w248]
      disable-tunnel: w162 -> [w238 w246]
      frame Enabled {
        w239 = refnum<k21> "PXIe_DStarC" ("FPGA I/O In")
        # "Do not remove\nHandles trigger hold-off"
        # "Configure mmWave Port - re-use trig 6"
        # "Pass-through resource"
        # "Arbitration is only required when using Trig 6, other triggers can be accessed normally. Trig 4 is reserved for runtime synchronization"
        n101 = call <instrlib>:"Configure mmWave Port.vi"("port"=w242, "pxi trigger"=w239, "input valid"=w243) -> ()  [unwired: 12 in, 1 out]
        n102 = xnode "FPGA I/O Node"("FPGA I/O In"=w239) -> ("I/O Item"=w241:bool)  [unwired: 1 out]
        n103 = Bundle By Name(cluster=T28 {"disable TClk measure"=FALSE, "output enable"=FALSE, "output value"=FALSE} ("pxi trig 6 arbiter"), "output enable"=w240, "output value"=w241, "disable TClk measure"=w238) -> (w244:T28)
        n104 = global write "Globals.vi" "pxi trig 6 arbiter"(w244) -> ()
      }
      frame Disabled {
        w250 = FALSE ("disable TClk measure")
        # "Note: this configuration is preferred but \nuses an additional trigger line"
        # "Configure mmWave Port - dedicated trigger"
        # "Arbitration is only required when using Trig 6, other triggers can be accessed normally. Trig 4 is reserved for runtime synchronization"
        n105 = xnode "FPGA I/O Method Node"("FPGA I/O In"=refnum<k21> "PXI_Trig0" ("pxi trigger 1"), "Enable"=w248) -> ("FPGA I/O Out"=w249:refnum<k21>)
        n106 = call <instrlib>:"Configure mmWave Port.vi"("port"=w251, "pxi trigger"=w249, "input valid"=w252) -> ()  [unwired: 12 in, 1 out]
        n107 = Bundle By Name(cluster=T28 {"disable TClk measure"=FALSE, "output enable"=FALSE, "output value"=FALSE} ("pxi trig 6 arbiter"), "output enable"=w250, "output value"=w250, "disable TClk measure"=w246) -> (w253:T28)
        n108 = global write "Globals.vi" "pxi trig 6 arbiter"(w253) -> ()
      }
    }
    n109 = global read "Globals.vi" "rxjesd.control"() -> (w188:T11)
    n110 = Build Array (concatenate)(w124, w121) -> (w122:bool[])
    n111 = Array Subset(array=w122, length=384) -> (w120:bool[])  [unwired: 1 in]
    n112 = call "RX JESD.vi"("rxjesd.control"=w188) -> ("trigger output enable"=w152:bool, "trigger value"=w172:bool)  [unwired: 13 in]
    n113 = Compound Arithmetic op=AND("gain ranging.enable coarse gain ranging", invert "sync.master reset listen") -> (w160:bool)
    n114 = feedback #13(bool[] [FALSE, FALSE, FALSE, FALSE, FALSE, FALSE, FALSE, FALSE, FALSE, FALSE, FALSE, FALSE, FALSE, FALSE, FALSE, FALSE, FALSE, FALSE, FALSE, FALSE, FALSE, FALSE, FALSE, FALSE, FALSE, FALSE, FALSE, FALSE, FALSE, FALSE, FALSE, FALSE, FALSE, FALSE, FALSE, FALSE, FALSE, FALSE, FALSE, FALSE, FALSE, FALSE, FALSE, FALSE, FALSE, FALSE, FALSE, FALSE, FALSE, FALSE, FALSE, FALSE, FALSE, FALSE, FALSE, FALSE, FALSE, FALSE, FALSE, FALSE, FALSE, FALSE, FALSE, FALSE, FALSE, FALSE, FALSE, FALSE, FALSE, FALSE, FALSE, FALSE, FALSE, FALSE, FALSE, FALSE, FALSE, FALSE, FALSE, FALSE, FALSE, FALSE, FALSE, FALSE, FALSE, FALSE, FALSE, FALSE, FALSE, FALSE, FALSE, FALSE, FALSE, FALSE, FALSE, FALSE, FALSE, FALSE, FALSE, FALSE, FALSE, FALSE, FALSE, FALSE, FALSE, FALSE, FALSE, FALSE, FALSE, FALSE, FALSE, FALSE, FALSE, FALSE, FALSE, FALSE, FALSE, FALSE, FALSE, FALSE, FALSE, FALSE, FALSE, FALSE, FALSE, FALSE, FALSE, FALSE, FALSE, FALSE, FALSE, FALSE, FALSE, FALSE, FALSE, FALSE, FALSE, FALSE, FALSE, FALSE, FALSE, FALSE, FALSE, FALSE, FALSE, FALSE, FALSE, FALSE, FALSE, FALSE, FALSE, FALSE, FALSE, FALSE, FALSE, FALSE, FALSE, FALSE, FALSE, FALSE, FALSE, FALSE, FALSE, FALSE, FALSE, FALSE, FALSE, FALSE, FALSE, FALSE, FALSE, FALSE, FALSE, FALSE, FALSE, FALSE, FALSE, FALSE, FALSE, FALSE, FALSE, FALSE, FALSE, FALSE, FALSE, FALSE, FALSE, FALSE, FALSE, FALSE, FALSE, FALSE, FALSE, FALSE, FALSE, FALSE, FALSE, FALSE, FALSE, FALSE, FALSE, FALSE, FALSE, FALSE, FALSE, FALSE, FALSE, FALSE, FALSE, FALSE, FALSE, FALSE, FALSE, FALSE, FALSE, FALSE, FALSE, FALSE, FALSE, FALSE, FALSE, FALSE, FALSE, FALSE, FALSE, FALSE, FALSE, FALSE, FALSE, FALSE, FALSE, FALSE, FALSE, FALSE, FALSE, FALSE, FALSE, FALSE, FALSE, FALSE, FALSE, FALSE, FALSE, FALSE, FALSE, FALSE, FALSE, FALSE, FALSE, FALSE, FALSE, FALSE, FALSE, FALSE, FALSE, FALSE, FALSE, FALSE, FALSE, FALSE, FALSE, FALSE, FALSE, FALSE, FALSE, FALSE, FALSE, FALSE, FALSE, FALSE, FALSE, FALSE, FALSE, FALSE, FALSE, FALSE, FALSE, FALSE, FALSE, FALSE, FALSE, FALSE, FALSE, FALSE, FALSE, FALSE, FALSE, FALSE, FALSE, FALSE, FALSE, FALSE, FALSE, FALSE, FALSE, FALSE, FALSE, FALSE, FALSE, FALSE, FALSE, FALSE, FALSE, FALSE, FALSE, FALSE, FALSE, FALSE, FALSE, FALSE, FALSE, FALSE, FALSE, FALSE, FALSE, FALSE, FALSE, FALSE, FALSE, FALSE, FALSE, FALSE, FALSE, FALSE, FALSE, FALSE, FALSE, FALSE, FALSE, FALSE, FALSE, FALSE, FALSE, FALSE, FALSE, FALSE, FALSE, FALSE, FALSE, FALSE, FALSE, FALSE, FALSE, FALSE, FALSE, FALSE, FALSE, FALSE, FALSE, FALSE, FALSE, FALSE, FALSE, FALSE, FALSE, FALSE, FALSE, FALSE, FALSE, FALSE, FALSE, FALSE, FALSE, FALSE, FALSE, FALSE, FALSE, FALSE, FALSE, FALSE, FALSE, FALSE, FALSE, FALSE, FALSE, FALSE, FALSE, FALSE, FALSE, FALSE, FALSE, FALSE, FALSE, FALSE]) -> (w111:bool[])
    n115 = feedback-in #13(w120) -> ()
    n116 = Or(x=w152, y="gain ranging.enable coarse gain ranging") -> (x .or. y?=w168:bool)
    n117 = call-poly <instrlib>:"Count Down.vi"("count in"="acq.length", "load"=w200, "decrement"=w109) -> ("terminal count"=w198:bool)  [unwired: 11 in, 1 out]
    n118 = call <instrlib>:"Synchronous Latch.vi"("clear"=w198, "set"=w200) -> ("out"=w199:bool)  [unwired: 9 in]
    n119 = feedback-in #12(w199) -> ()
    n120 = call <instrlib>:"Write gain setting (Fine).vi"("gain"=w185, "table info"="table info", "P2P Writer FIFO"=refnum<k21> "P2P FIFO to PXIe-3620" ("FIFO In"), "direction"=enum8{"rx", "tx"}."rx", "input valid"=w180) -> ()  [unwired: 10 in, 1 out]
    n121 = call-poly <instrlib>:"Packer.vi"("data in"=w111, "reset"=w100, "DRAM FIFO in"=w110, "flush data"="dram.flush", "input valid"=w109) -> ("data out"=w116:bool[], "output valid"=w117:bool)  [unwired: 8 in, 1 out]
    n122 = Or(x="sync.master reset listen", y=w152) -> (x .or. y?=w151:bool)
    n123 = xnode "FPGA I/O Method Node"("FPGA I/O In"=refnum<k21> "PXI_Trig5" ("pxi trigger 1"), "Enable"=w168) -> ("FPGA I/O Out"=w171:refnum<k21>)
    n124 = xnode "FPGA I/O Method Node"("FPGA I/O In"=refnum<k21> "PXI_Trig7" ("pxi trigger 1"), "Enable"=w160) -> ("FPGA I/O Out"=w173:refnum<k21>)
    n125 = feedback #14(bool[] [FALSE, FALSE, FALSE, FALSE, FALSE, FALSE, FALSE, FALSE, FALSE, FALSE, FALSE, FALSE, FALSE, FALSE, FALSE, FALSE, FALSE, FALSE, FALSE, FALSE, FALSE, FALSE, FALSE, FALSE, FALSE, FALSE, FALSE, FALSE, FALSE, FALSE, FALSE, FALSE, FALSE, FALSE, FALSE, FALSE, FALSE, FALSE, FALSE, FALSE, FALSE, FALSE, FALSE, FALSE, FALSE, FALSE, FALSE, FALSE, FALSE, FALSE, FALSE, FALSE, FALSE, FALSE, FALSE, FALSE, FALSE, FALSE, FALSE, FALSE, FALSE, FALSE, FALSE, FALSE, FALSE, FALSE, FALSE, FALSE, FALSE, FALSE, FALSE, FALSE, FALSE, FALSE, FALSE, FALSE, FALSE, FALSE, FALSE, FALSE, FALSE, FALSE, FALSE, FALSE, FALSE, FALSE, FALSE, FALSE, FALSE, FALSE, FALSE, FALSE, FALSE, FALSE, FALSE, FALSE, FALSE, FALSE, FALSE, FALSE, FALSE, FALSE, FALSE, FALSE, FALSE, FALSE, FALSE, FALSE, FALSE, FALSE, FALSE, FALSE, FALSE, FALSE, FALSE, FALSE, FALSE, FALSE, FALSE, FALSE, FALSE, FALSE, FALSE, FALSE, FALSE, FALSE, FALSE, FALSE, FALSE, FALSE, FALSE, FALSE, FALSE, FALSE, FALSE, FALSE, FALSE, FALSE, FALSE, FALSE, FALSE, FALSE, FALSE, FALSE, FALSE, FALSE, FALSE, FALSE, FALSE, FALSE, FALSE, FALSE, FALSE, FALSE, FALSE, FALSE, FALSE, FALSE, FALSE, FALSE, FALSE, FALSE, FALSE, FALSE, FALSE, FALSE, FALSE, FALSE, FALSE, FALSE, FALSE, FALSE, FALSE, FALSE, FALSE, FALSE, FALSE, FALSE, FALSE, FALSE, FALSE, FALSE, FALSE, FALSE, FALSE, FALSE, FALSE, FALSE, FALSE, FALSE, FALSE, FALSE, FALSE, FALSE, FALSE, FALSE, FALSE, FALSE, FALSE, FALSE, FALSE, FALSE, FALSE, FALSE, FALSE, FALSE, FALSE, FALSE, FALSE, FALSE, FALSE, FALSE, FALSE, FALSE, FALSE, FALSE, FALSE, FALSE, FALSE, FALSE, FALSE, FALSE, FALSE, FALSE, FALSE, FALSE, FALSE, FALSE, FALSE, FALSE, FALSE, FALSE, FALSE, FALSE, FALSE, FALSE, FALSE, FALSE, FALSE, FALSE, FALSE, FALSE, FALSE, FALSE, FALSE, FALSE, FALSE, FALSE, FALSE, FALSE, FALSE, FALSE, FALSE, FALSE, FALSE, FALSE, FALSE, FALSE, FALSE, FALSE, FALSE, FALSE, FALSE, FALSE, FALSE, FALSE, FALSE, FALSE, FALSE, FALSE, FALSE, FALSE, FALSE, FALSE, FALSE, FALSE, FALSE, FALSE, FALSE, FALSE, FALSE, FALSE, FALSE, FALSE, FALSE, FALSE, FALSE, FALSE, FALSE, FALSE, FALSE, FALSE, FALSE, FALSE, FALSE, FALSE, FALSE, FALSE, FALSE, FALSE, FALSE, FALSE, FALSE, FALSE, FALSE, FALSE, FALSE, FALSE, FALSE, FALSE, FALSE, FALSE, FALSE, FALSE, FALSE, FALSE, FALSE, FALSE, FALSE, FALSE, FALSE, FALSE, FALSE, FALSE, FALSE, FALSE, FALSE, FALSE, FALSE, FALSE, FALSE, FALSE, FALSE, FALSE, FALSE, FALSE, FALSE, FALSE, FALSE, FALSE, FALSE, FALSE, FALSE, FALSE, FALSE, FALSE, FALSE, FALSE, FALSE, FALSE, FALSE, FALSE, FALSE, FALSE, FALSE, FALSE, FALSE, FALSE, FALSE, FALSE, FALSE, FALSE, FALSE, FALSE, FALSE, FALSE, FALSE, FALSE, FALSE, FALSE, FALSE, FALSE, FALSE, FALSE, FALSE, FALSE, FALSE, FALSE, FALSE, FALSE, FALSE, FALSE, FALSE, FALSE, FALSE, FALSE, FALSE, FALSE, FALSE, FALSE, FALSE, FALSE, FALSE, FALSE, FALSE, FALSE, FALSE, FALSE, FALSE, FALSE, FALSE, FALSE, FALSE, FALSE, FALSE, FALSE, FALSE, FALSE, FALSE, FALSE, FALSE, FALSE, FALSE, FALSE, FALSE, FALSE, FALSE, FALSE, FALSE, FALSE, FALSE, FALSE, FALSE, FALSE, FALSE, FALSE, FALSE, FALSE, FALSE, FALSE, FALSE, FALSE, FALSE, FALSE, FALSE, FALSE, FALSE, FALSE, FALSE, FALSE, FALSE, FALSE, FALSE, FALSE, FALSE, FALSE, FALSE, FALSE, FALSE, FALSE, FALSE, FALSE, FALSE, FALSE, FALSE, FALSE, FALSE, FALSE, FALSE, FALSE, FALSE, FALSE, FALSE, FALSE, FALSE, FALSE, FALSE, FALSE, FALSE, FALSE, FALSE, FALSE, FALSE, FALSE, FALSE, FALSE, FALSE, FALSE, FALSE, FALSE, FALSE, FALSE, FALSE, FALSE, FALSE, FALSE, FALSE, FALSE, FALSE, FALSE, FALSE, FALSE, FALSE, FALSE, FALSE, FALSE, FALSE, FALSE, FALSE, FALSE, FALSE, FALSE, FALSE, FALSE, FALSE, FALSE, FALSE, FALSE, FALSE, FALSE, FALSE, FALSE]) -> (w102:bool[])
    n126 = feedback-in #14(w116) -> ()
    n127 = feedback #15() -> (w101:bool)  [unwired: 1 in]
    n128 = feedback-in #15(w117) -> ()
    n129 = call <instrlib>:"Write.vi"("element"=w102, "DRAM FIFO ref in"=w110, "input valid"=w101) -> ("ready for input"=w115:bool)  [unwired: 12 in]
    n130 = Not(x=w115) -> (.not. x?=w114:bool)
    n131 = call <instrlib>:"Synchronous Latch.vi"("clear"=w100, "set"=w114) -> ("out"=→"dram.overflow":bool)  [unwired: 9 in]
    n132 = case shown="True" w151 {
      tunnel: w173 -> [w226 w227]
      tunnel: w172 -> [_ w231]
      tunnel: w171 -> [w225 w230]
      tunnel: w170 -> [w224 _]
      tunnel: w169 -> [w223 _]
      tunnel: [FALSE ("Master10k_Reset") w229] -> w157
      tunnel: "sync.master reset listen" -> [_ w228]
      frame False {
        # "Gain Ranging - not required"
        n133 = call <instrlib>:"Write gain setting (Coarse).vi"("fast jump table index"=w224, "pxi trigger 1"=w225, "pxi trigger 2"=w226, "input valid"=w223) -> ()  [unwired: 11 in, 1 out]
      }
      frame True {
        # "Rx JESD Sync - required"
        n134 = case shown="True" w228 {
          tunnel: w231 -> [w234 _]
          tunnel: w230 -> [w233 _]
          tunnel: [FALSE ("Master10k_Reset") w235] -> w229
          tunnel: w227 -> [_ w236]
          frame False {
            n135 = xnode "FPGA I/O Method Node"("FPGA I/O In"=w233, "Data"=w234) -> ()  [unwired: 1 out]
          }
          frame True {
            # "Receive master 10 kHz reset"
            n136 = xnode "FPGA I/O Node"("FPGA I/O In"=w236) -> ("I/O Item"=w237:bool)  [unwired: 1 out]
            n137 = call "Master 10 kHz Reset.vi"("I/O Item"=w237) -> ("master 10 kHz reset"=w235:bool)  [unwired: 10 in]
          }
        }
      }
    }
    n138 = And(x="sync.counter reset enable", y=w157) -> (x .and. y?=w156:bool)
    n139 = feedback-in #10(w156) -> ()
  }
  n140 = node-c288() -> (w37:T23)  [unwired: 1 in]
  n141 = timed-loop {
    timing: w37 -> [_]
    timing-out: [_] -> w36
    tunnel: w34 -> [w271]
    tunnel: w33 -> [w270]
    tunnel: w29 -> [w265]
    tunnel: w30 -> [w266]
    tunnel: w27 -> [w263]
    tunnel: w19 -> [w261]
    tunnel: w20 -> [w262]
    stop <- _ stop-if-true
    n142 = call "Get Clock State.vi"("handshake in"=w271) -> ("clock valid"=w269:bool)  [unwired: 14 in]
    n143 = call "Get Clock State.vi"("handshake in"=w270) -> ("clock valid"=w268:bool)  [unwired: 14 in]
    n144 = call "Get Clock State.vi"("handshake in"=w265) -> ("clock valid"=w264:bool)  [unwired: 14 in]
    n145 = call "Get Clock State.vi"("handshake in"=w261) -> ("clock valid"=w258:bool)  [unwired: 14 in]
    n146 = call "Get Clock State.vi"("handshake in"=w262) -> ("clock valid"=w257:bool)  [unwired: 14 in]
    n147 = call "Get Clock State.vi"("handshake in"=w266) -> ("clock valid"=w259:bool)  [unwired: 14 in]
    n148 = call "Get Clock State.vi"("handshake in"=w263) -> ("clock valid"=w260:bool)  [unwired: 14 in]
    n149 = Build Array(w269, w268, w264, w258, w257, w259, w260) -> (→"clocks valid":bool[])
  }
  n150 = node-c288(w36) -> ()
  n151 = node-c288(w7) -> ()
  n152 = node-c288() -> (w42:T23)  [unwired: 1 in]
  n153 = timed-loop {
    timing: w42 -> [_]
    timing-out: [_] -> w41
    stop <- _ stop-if-true
    # "CLIP Control and Status"
    n154 = Unbundle By Name("rxjesd.control") -> ("gtx enable"=w276:bool, "jesd enable"=w280:bool, "sw sync"=w279:bool, "buffer enable"=w278:bool, "clock enable"=w275:bool)
    n155 = global write "Globals.vi" "rxjesd.control"("rxjesd.control") -> ()
    n156 = xnode "FPGA I/O Node"("7902R IO Socket\\aGtxEnable"=w276, "7902R IO Socket\\aJesdEnable"=w280, "7902R IO Socket\\aSyncFromSw"=w279, "7902R IO Socket\\aBufferEnable"=w278, "7902R IO Socket\\aClkEnable"=w275) -> ()  [unwired: 5 in, 5 out]
    n157 = xnode "FPGA I/O Node"() -> ("7902R IO Socket\\aGtxActive"=w274:bool, "7902R IO Socket\\aJesdActive"=w297:bool, "7902R IO Socket\\aLaneSyncReq"=w296:bool, "7902R IO Socket\\aLanesSynced"=w295:bool, "7902R IO Socket\\aLanesAligned"=w294:bool, "7902R IO Socket\\aQpllLocked"=w293:bool, "7902R IO Socket\\aQpllRefLost"=w292:bool, "7902R IO Socket\\aKCharError"=w291:bool, "7902R IO Socket\\aLaneAlignError"=w290:bool, "7902R IO Socket\\a8b10bNotInTable"=w289:bool, "7902R IO Socket\\a8b10bDispError"=w288:bool, "7902R IO Socket\\aBufferOverflow"=w287:bool, "7902R IO Socket\\aBufferUnderflow"=w286:bool, "7902R IO Socket\\aBufferReady"=w285:bool, "7902R IO Socket\\MgtRefClks_Locked"=w284:bool, "7902R IO Socket\\MgtRefClks_Valid"=w283:bool, "7902R IO Socket\\sFrontEndConfig_Complete"=w282:bool)  [unwired: 17 in, 17 out]
    n158 = Bundle By Name(cluster=T12 {"gtx active"=FALSE, "jesd active"=FALSE, "lane sync req"=FALSE, "lanes synced"=FALSE, "lanes aligned"=FALSE, "qpll locked"=FALSE, "qpll ref lost"=FALSE, "k-char error"=FALSE, "lane alignment error"=FALSE, "8b10b error"=FALSE, "8b10b disparity error"=FALSE, "buffer overflow"=FALSE, "buffer underflow"=FALSE, "buffer ready"=FALSE, "mgt ref clocks locked"=FALSE, "mgt ref clock valid"=FALSE, "config complete"=FALSE} ("rxjesd.status 2"), "gtx active"=w274, "jesd active"=w297, "lane sync req"=w296, "lanes synced"=w295, "lanes aligned"=w294, "qpll locked"=w293, "qpll ref lost"=w292, "k-char error"=w291, "lane alignment error"=w290, "8b10b error"=w289, "8b10b disparity error"=w288, "buffer overflow"=w287, "buffer underflow"=w286, "buffer ready"=w285, "mgt ref clocks locked"=w284, "mgt ref clock valid"=w283, "config complete"=w282) -> (→"rxjesd.status":T12)
  }
  n159 = node-c288(w4) -> ()
  n160 = call "Aurora Create Resources (Single Port).vi"("RX CLIP Resources"=T21 {"m_axis_tvalid"="7902R IO Socket\\uPort5_m_axi_rx_tvalid", "m_axis_tdata_0"="7902R IO Socket\\uPort5_m_axi_rx_tdata_0", "m_axis_tdata_1"="7902R IO Socket\\uPort5_m_axi_rx_tdata_1", "m_axis_tdata_2"="7902R IO Socket\\uPort5_m_axi_rx_tdata_2", "m_axis_tdata_3"="7902R IO Socket\\uPort5_m_axi_rx_tdata_3"}, "TX CLIP Resources"=T22 {"s_axis_tvalid"="7902R IO Socket\\uPort5_s_axi_tx_tvalid", "s_axis_tdata_0"="7902R IO Socket\\uPort5_s_axi_tx_tdata_0", "s_axis_tdata_1"="7902R IO Socket\\uPort5_s_axi_tx_tdata_1", "s_axis_tdata_2"="7902R IO Socket\\uPort5_s_axi_tx_tdata_2", "s_axis_tdata_3"="7902R IO Socket\\uPort5_s_axi_tx_tdata_3", "s_axis_tready"="7902R IO Socket\\uPort5_s_axi_tx_tready"}) -> ("AXI4-Stream Reader FXP64x4"=w12:T30, "AXI4-Stream Writer FXP64x4"=w13:T31)  [unwired: 8 in]
  n161 = call "Aurora Create Resources (Single Port).vi"("RX CLIP Resources"=T21 {"m_axis_tvalid"="7902R IO Socket\\uPort4_m_axi_rx_tvalid", "m_axis_tdata_0"="7902R IO Socket\\uPort4_m_axi_rx_tdata_0", "m_axis_tdata_1"="7902R IO Socket\\uPort4_m_axi_rx_tdata_1", "m_axis_tdata_2"="7902R IO Socket\\uPort4_m_axi_rx_tdata_2", "m_axis_tdata_3"="7902R IO Socket\\uPort4_m_axi_rx_tdata_3"}, "TX CLIP Resources"=T22 {"s_axis_tvalid"="7902R IO Socket\\uPort4_s_axi_tx_tvalid", "s_axis_tdata_0"="7902R IO Socket\\uPort4_s_axi_tx_tdata_0", "s_axis_tdata_1"="7902R IO Socket\\uPort4_s_axi_tx_tdata_1", "s_axis_tdata_2"="7902R IO Socket\\uPort4_s_axi_tx_tdata_2", "s_axis_tdata_3"="7902R IO Socket\\uPort4_s_axi_tx_tdata_3", "s_axis_tready"="7902R IO Socket\\uPort4_s_axi_tx_tready"}) -> ("AXI4-Stream Reader FXP64x4"=w10:T30, "AXI4-Stream Writer FXP64x4"=w11:T31)  [unwired: 8 in]
  n162 = node-c288 ("Input Node")() -> (w15:T23)  [unwired: 1 in]
  n163 = node-c288() -> (w17:T23)  [unwired: 1 in]
  n164 = timed-loop {
    timing: w15 -> [_]
    timing-out: [_] -> w14
    tunnel: w13 -> [w306]
    tunnel: w12 -> [w310]
    stop <- _ stop-if-true
    # "Aurora read cannot be arbitrated. This must be true or left unwired.\n\nUse aurora.read port control for lossy post-read arbitration."
    # "Aurora read is disabled in this reference\nexample.  If enabled, a FIFO reader must\nbe provided."
    # "Single Port - 5.5GB/s"
    n165 = call "Aurora Reader (Single Port) .vi"("AXI4-Stream Reader FXP64x4"=w310, "ready for output"=TRUE) -> ("data"=w311:bool[], "output valid"=w304:bool)  [unwired: 12 in]
    n166 = And(x=w304, y="aurora.read port 5") -> (x .and. y?=w302:bool)
    n167 = case shown="True" w302 {
      tunnel: w311 -> [_ w329]
      tunnel: [FALSE ("Timed Out?") w328] -> w305
      frame False {
      }
      frame True {
        n168 = disable-structure shown="Disabled" {
          disable-tunnel: w329 -> [w332 _]
          disable-tunnel: [w331 _] -> w328
          frame Disabled {
            n169 = xnode ("FIFO Method Node")("Element"=w332, "Timeout"=0) -> ("Timed Out?"=w331:bool)  [unwired: 1 in, 1 out]
          }
          frame Enabled {
          }
        }
      }
    }
    n170 = call <instrlib>:"Synchronous Latch.vi"("clear"="port 5.rx fifo overflow clear", "set"=w305) -> ("out"=→"port 5.rx fifo overflow":bool)  [unwired: 9 in]
    n171 = feedback #16(FALSE ("ready for input")) -> (w313:bool)
    n172 = case shown="True" w313 {
      tunnel: [_ w321] -> w309
      tunnel: [TRUE ("Timed Out?") w320] -> w314
      frame False {
      }
      frame True {
        n173 = disable-structure shown="Enabled" {
          disable-tunnel: [w324 bool[] [FALSE, FALSE, FALSE, FALSE, FALSE, FALSE, FALSE, FALSE, FALSE, FALSE, FALSE, FALSE, FALSE, FALSE, FALSE, FALSE, FALSE, FALSE, FALSE, FALSE, FALSE, FALSE, FALSE, FALSE, FALSE, FALSE, FALSE, FALSE, FALSE, FALSE, FALSE, FALSE, FALSE, FALSE, FALSE, FALSE, FALSE, FALSE, FALSE, FALSE, FALSE, FALSE, FALSE, FALSE, FALSE, FALSE, FALSE, FALSE, FALSE, FALSE, FALSE, FALSE, FALSE, FALSE, FALSE, FALSE, FALSE, FALSE, FALSE, FALSE, FALSE, FALSE, FALSE, FALSE, FALSE, FALSE, FALSE, FALSE, FALSE, FALSE, FALSE, FALSE, FALSE, FALSE, FALSE, FALSE, FALSE, FALSE, FALSE, FALSE, FALSE, FALSE, FALSE, FALSE, FALSE, FALSE, FALSE, FALSE, FALSE, FALSE, FALSE, FALSE, FALSE, FALSE, FALSE, FALSE, FALSE, FALSE, FALSE, FALSE, FALSE, FALSE, FALSE, FALSE, FALSE, FALSE, FALSE, FALSE, FALSE, FALSE, FALSE, FALSE, FALSE, FALSE, FALSE, FALSE, FALSE, FALSE, FALSE, FALSE, FALSE, FALSE, FALSE, FALSE, FALSE, FALSE, FALSE, FALSE, FALSE, FALSE, FALSE, FALSE, FALSE, FALSE, FALSE, FALSE, FALSE, FALSE, FALSE, FALSE, FALSE, FALSE, FALSE, FALSE, FALSE, FALSE, FALSE, FALSE, FALSE, FALSE, FALSE, FALSE, FALSE, FALSE, FALSE, FALSE, FALSE, FALSE, FALSE, FALSE, FALSE, FALSE, FALSE, FALSE, FALSE, FALSE, FALSE, FALSE, FALSE, FALSE, FALSE, FALSE, FALSE, FALSE, FALSE, FALSE, FALSE, FALSE, FALSE, FALSE, FALSE, FALSE, FALSE, FALSE, FALSE, FALSE, FALSE, FALSE, FALSE, FALSE, FALSE, FALSE, FALSE, FALSE, FALSE, FALSE, FALSE, FALSE, FALSE, FALSE, FALSE, FALSE, FALSE, FALSE, FALSE, FALSE, FALSE, FALSE, FALSE, FALSE, FALSE, FALSE, FALSE, FALSE, FALSE, FALSE, FALSE, FALSE, FALSE, FALSE, FALSE, FALSE, FALSE, FALSE, FALSE, FALSE, FALSE, FALSE, FALSE, FALSE, FALSE, FALSE, FALSE, FALSE, FALSE, FALSE, FALSE, FALSE, FALSE, FALSE, FALSE, FALSE, FALSE, FALSE, FALSE, FALSE, FALSE, FALSE, FALSE, FALSE, FALSE, FALSE, FALSE, FALSE, FALSE, FALSE] ("Element")] -> w321
          disable-tunnel: [w323 TRUE ("Timed Out?")] -> w320
          frame Disabled {
            n174 = xnode ("FIFO Method Node")("Timeout"=0) -> ("Element"=w324:bool[], "Timed Out?"=w323:bool)  [unwired: 1 in, 1 out]
          }
          frame Enabled {
          }
        }
      }
    }
    n175 = call "Aurora Read Debug Signals (Single Port).vi"("Debug CLIP Resources"=T32 {"Hard Error"="7902R IO Socket\\uPort5_HardError", "Soft Error"="7902R IO Socket\\uPort5_SoftError", "Lane Up"="7902R IO Socket\\uPort5_LaneUp", "Channel Up"="7902R IO Socket\\uPort5_ChannelUp", "Sys Reset"="7902R IO Socket\\uPort5_sys_reset_out"}) -> ("Debug Info"=→"port 5.debug info":T5)  [unwired: 14 in]
    n176 = Not(x=w314) -> (.not. x?=w308:bool)
    n177 = call "Aurora Writer (Single Port).vi"("input data"=w309, "AXI4-Stream Writer FXP64x4"=w306, "input valid"=w308) -> ("ready for input"=w307:bool)  [unwired: 12 in]
    n178 = feedback-in #16(w307) -> ()
  }
  n179 = timed-loop {
    timing: w17 -> [_]
    timing-out: [_] -> w16
    tunnel: w11 -> [w352]
    tunnel: w10 -> [w338]
    stop <- _ stop-if-true
    # "Aurora read cannot be arbitrated. This must be true or left unwired.\n\nUse aurora.read port control for lossy post-read arbitration."
    # "Single Port - 5.5GB/s"
    n180 = call "Aurora Reader (Single Port) .vi"("AXI4-Stream Reader FXP64x4"=w338, "ready for output"=TRUE) -> ("data"=w339:bool[], "output valid"=w340:bool)  [unwired: 12 in]
    n181 = And(x=w340, y="aurora.read port 4") -> (x .and. y?=w335:bool)
    n182 = disable-structure shown="Enabled" {
      disable-tunnel: w339 -> [w354 _]
      disable-tunnel: [w355 _] -> w337
      disable-tunnel: w335 -> [w353 _]
      frame Enabled {
        n183 = xnode ("FIFO Write Using Handshaking")("Element"=w354, "Input Valid"=w353) -> ("Ready for Input"=w356:bool)  [unwired: 1 in, 1 out]
        n184 = Not(x=w356) -> (.not. x?=w355:bool)
      }
      frame Disabled {
      }
    }
    n185 = call <instrlib>:"Synchronous Latch.vi"("clear"="port 4.rx fifo overflow clear", "set"=w337) -> ("out"=→"port 4.rx fifo overflow":bool)  [unwired: 9 in]
    n186 = feedback #17(FALSE ("ready for input")) -> (w345:bool)
    n187 = case shown="True" w345 {
      tunnel: [_ w359] -> w351
      tunnel: [TRUE ("Timed Out?") w358] -> w348
      frame False {
      }
      frame True {
        n188 = disable-structure shown="Enabled" {
          disable-tunnel: [w362 _] -> w359
          disable-tunnel: [w361 TRUE ("Timed Out?")] -> w358
          frame Enabled {
            n189 = xnode ("FIFO Method Node")("Timeout"=0) -> ("Element"=w362:bool[], "Timed Out?"=w361:bool)  [unwired: 1 in, 1 out]
          }
          frame Disabled {
          }
        }
      }
    }
    n190 = call "Aurora Read Debug Signals (Single Port).vi"("Debug CLIP Resources"=T32 {"Hard Error"="7902R IO Socket\\uPort4_HardError", "Soft Error"="7902R IO Socket\\uPort4_SoftError", "Lane Up"="7902R IO Socket\\uPort4_LaneUp", "Channel Up"="7902R IO Socket\\uPort4_ChannelUp", "Sys Reset"="7902R IO Socket\\uPort4_sys_reset_out"}) -> ("Debug Info"=→"port 4.debug info":T5)  [unwired: 14 in]
    n191 = Not(x=w348) -> (.not. x?=w347:bool)
    n192 = call "Aurora Writer (Single Port).vi"("input data"=w351, "AXI4-Stream Writer FXP64x4"=w352, "input valid"=w347) -> ("ready for input"=w346:bool)  [unwired: 12 in]
    n193 = feedback-in #17(w346) -> ()
  }
  n194 = node-c288(w41) -> ()
  n195 = node-c288(w16) -> ()
  n196 = node-c288(w14) -> ()
  n197 = node-c288(w39) -> ()
